vi "Main_PotentialField.vi"() -> ()   [LabVIEW 2019]
uses:
  Ctrl/cmd_common.ctl
panel:
  in  "set-val":T1={"start pt"={"x"=0.0, "y"=10.0}, "goal pt"={"x"=30.0, "y"=30.0}, "grid size"=0.5, "robot radius"=5.0, "obstacles"=[{"x"=15.0, "y"=25.0}, {"x"=5.0, "y"=15.0}, {"x"=20.0, "y"=26.0}, {"x"=25.0, "y"=25.0}]}
  in  "global-val":T2={"KP"=5.0, "ETA"=100.0, "AREA_WIDTH"=30.0, "Osc_Det_Len"=3}
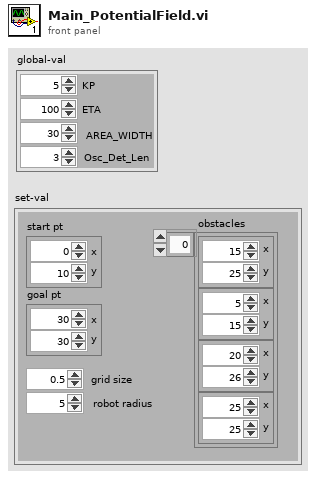
[diagram p1: front panel]
types:
  T1 = cluster{"start pt":cluster{"x":dbl, "y":dbl}, "goal pt":cluster{"x":dbl, "y":dbl}, "grid size":dbl, "robot radius":dbl, "obstacles":cluster{"x":dbl, "y":dbl}[]}
  T2 = cluster{"KP":dbl, "ETA":dbl, "AREA_WIDTH":dbl, "Osc_Det_Len":u32}
  T3 = typedef "cmd_common.ctl" = enum16{"read", "write"}
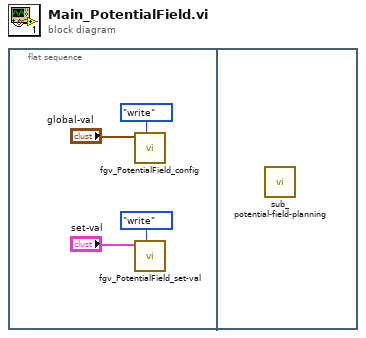
[diagram p0: block diagram]
diagram:
  n1 = flat-sequence {
    frame #0 {
      n2 = call "fgv_PotentialField_config.vi"("cmd"=cmd_common."write", "pf-val"="global-val") -> ()  [unwired: 9 in, 1 out]
      n3 = call "fgv_PotentialField_set-val.vi"("cmd"=cmd_common."write", "set-val"="set-val") -> ()  [unwired: 9 in, 1 out]
    }
    frame #1 {
      n4 = call "sub_potential-field-planning.vi"() -> ()  [unwired: 12 in]
    }
  }
